vi "DAQ_set_Shutters.vi"() -> ()   [LabVIEW 2015]
uses:
  <vilib>/DAQmx/write.llb/DAQmx Write.vi
  <vilib>/DAQmx/write.llb/DAQmx Write (Digital 1D Bool NChan 1Samp 1Line).vi
  <vilib>/DAQmx/miscellaneous.llb/DAQmx Fill In Error Info.vi
panel:
  out "error out":errorcluster
  in  "Channel Names In":string[](array[string])
  in  "Lines in":string[](array[string])
  in  "error in":errorcluster
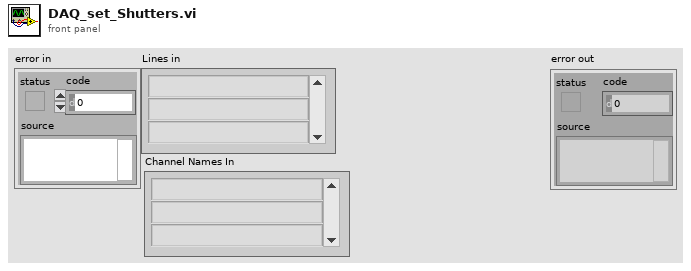
[diagram p1: front panel]
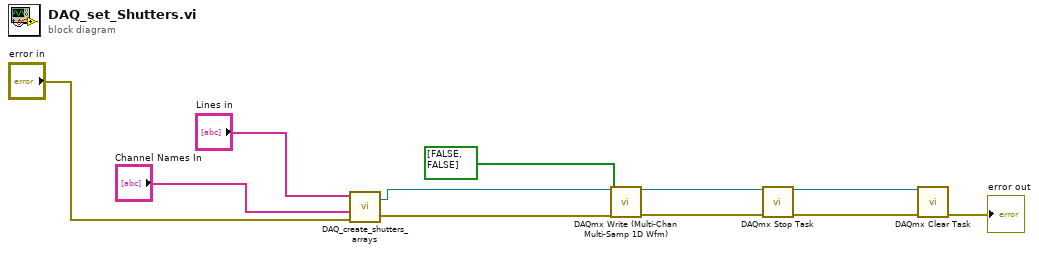
[diagram p0: block diagram]
diagram:
  n1 = call "DAQ_create_shutters_arrays.vi"("error in"="error in", "Channel Names In"="Channel Names In", "Lines in"="Lines in") -> ("error out"=w8:errorcluster, "task out"=w7:refnum<k21>)  [unwired: 1 in]
  n2 = call-poly "DAQmx Write (Multi-Chan Multi-Samp 1D Wfm).vi"("task/channels in"=w7, "data"=bool[] [FALSE, FALSE], "error in"=w8) -> ("task out"=w5:refnum<k21>, "error out"=w4:errorcluster)  [unwired: 10 in, 1 out]
  n3 = call <vilib>:"DAQmx Stop Task.vi"("task/channels in"=w5, "error in"=w4) -> ("task out"=w3:refnum<k21>, "error out"=w2:errorcluster)  [unwired: 12 in]
  n4 = call <vilib>:"DAQmx Clear Task.vi"("task in"=w3, "error in"=w2) -> ("error out"=→"error out":errorcluster)  [unwired: 13 in]
